vi "OE1022D_Configure_Acquisition.vi"(0 "VISA resource name":refnum<visa-resource-name>, 1 "OE1022D A/B":u8(ring) items=["Channel A", "Channel B"], 2 "Sample time (s)":dbl=0.001 min=0.001 max=100.0 step=0.001, 3 "error in (no error)":errorcluster, 7 "Sample Mode (Single/Loop)":u8(ring)=1 items=["Single", "Loop"]) -> (6 "VISA resource name out":refnum<visa-resource-name>, 9 "error out":errorcluster)   [LabVIEW 2022 SP3]
doc: "Configures the storage of the acquired data in the internal buffer.\n\n<B>Note:</B>\n\nThis VI configures how the data is acquired and stored from the display to the internal buffer of the instrument."
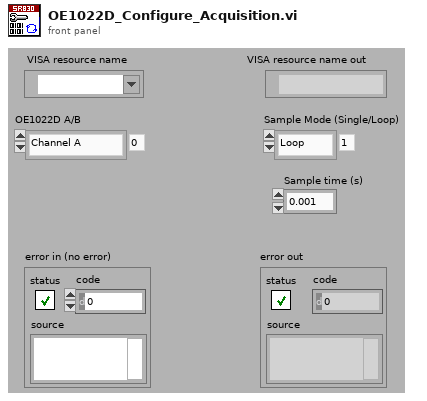
[diagram p1: front panel]
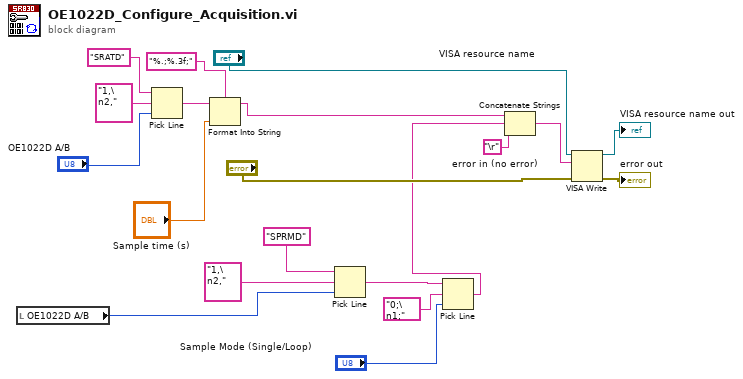
[diagram p0: block diagram]
diagram:
  n1 = local read "OE1022D A/B"() -> (w7:u8)
  n2 = Pick Line(string ("")="SRATD", multi-line string="1,\n2,", line index="OE1022D A/B") -> (output string=w14:string)
  n3 = Format Into String(format string="%.;%.3f;", initial string=w14, "Sample time (s)") -> (resulting string=w5:string)  [unwired: 1 in, 1 out]
  n4 = Pick Line(string ("")="SPRMD", multi-line string="1,\n2,", line index=w7) -> (output string=w4:string)
  n5 = Pick Line(string ("")=w4, multi-line string="0;\n1;", line index="Sample Mode (Single/Loop)") -> (output string=w1:string)
  n6 = Concatenate Strings(w5, w1, "\r") -> (w11:string)
  n7 = VISA Write(VISA resource name="VISA resource name", write buffer=w11, error in (no error)="error in (no error)") -> (VISA resource name out=→"VISA resource name out":refnum<visa-resource-name>, error out=→"error out":errorcluster)  [unwired: 1 out]
